vi "BeginService.vi"(1 "In":i32) -> (0 "Out":i32)   [LabVIEW 2011]
doc: "Copyright (c) 2005, Kuan Chen\nAll rights reserved.\n\nRedistribution and use in source and binary forms, with or without modification, are permitted provided that the following conditions are met:\n\n * Redistributions of source code must retain the above copyright notice, this list of conditions and the following disclaimer.\n * Redistributions in binary form must reproduce the above copyright notice, this list of conditions and the following disclaimer in the documentation and/or other materials provided with the distribution.\n * Neither the name of the Kuan Chen nor the names of its contributors may be used to endorse or promote products derived from this software without specific prior written permission.\n\nTHIS SOFTWARE IS PROVIDED BY THE COPYRIGHT HOLDERS AND CONTRIBUTORS \"AS IS\" AND ANY EXPRESS OR IMPLIED WARRANTIES, INCLUDING, BUT NOT LIMITED TO, THE IMPLIED WARRANTIES OF MERCHANTABILITY AND FITNESS FOR A PARTICULAR PURPOSE ARE DISCLAIMED. IN NO EVENT SHALL THE COPYRIGHT OWNER OR CONTRIBUTORS BE LIABLE FOR ANY DIRECT, INDIRECT, INCIDENTAL, SPECIAL, EXEMPLARY, OR CONSEQUENTIAL DAMAGES (INCLUDING, BUT NOT LIMITED TO, PROCUREMENT OF SUBSTITUTE GOODS OR SERVICES; LOSS OF USE, DATA, OR PROFITS; OR BUSINESS INTERRUPTION) HOWEVER CAUSED AND ON ANY THEORY OF LIABILITY, WHETHER IN CONTRACT, STRICT LIABILITY, OR TORT (INCLUDING NEGLIGENCE OR OTHERWISE) ARISING IN ANY WAY OUT OF THE USE OF THIS SOFTWARE, EVEN IF ADVISED OF THE POSSIBILITY OF SUCH DAMAGE.\n\nWrites a \"line n\" line to C:\\temp\\output.txt once per second, where n is the nth second. Stops when StopOutputThread.vi is used."
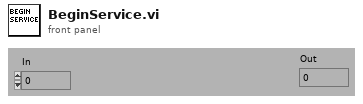
[diagram p1: front panel]
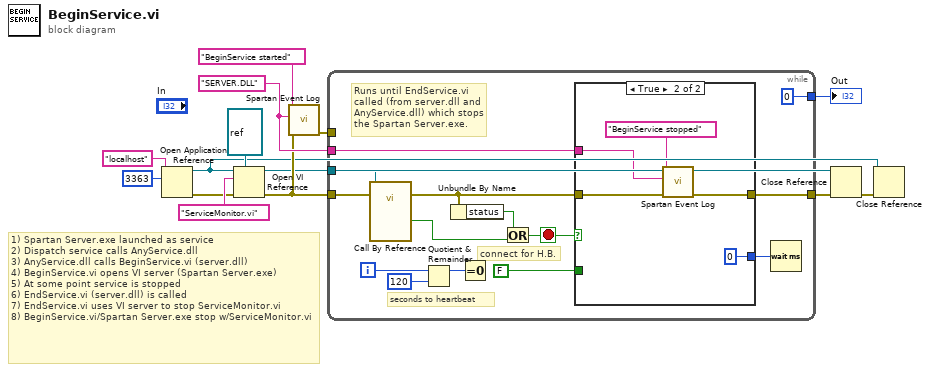
[diagram p0: block diagram]
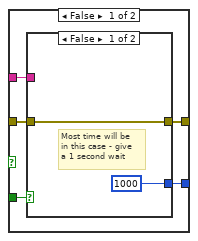
[diagram p2: hidden frame]
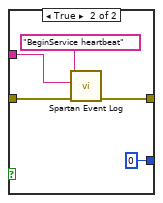
[diagram p3: hidden frame]
diagram:
  w12 = "SERVER.DLL" ("module (\"\")")
  # "1) Spartan Server.exe launched as service\n2) Dispatch service calls AnyService.dll\n3) AnyService.dll calls BeginService.vi (server.dll)\n4) BeginService.vi opens VI server (Spartan Server.exe)\n5) At some point service is stopped\n6) EndService.vi (server.dll) is called\n7) EndService.vi uses VI server to stop ServiceMonitor.vi\n8) BeginService.vi/Spartan Server.exe stop w/ServiceMonitor.vi"
  n1 = Open Application Reference(10:u16 3363 ("port number or service name (3363)"), 11:"localhost" ("machine name (\"\":  open local reference)")) -> (0:w5:errorcluster, 3:w3:refnum<vi>)  [unwired: 2 in]
  n2 = Open VI Reference(type specifier VI Refnum (for type only)=refnum<vi> refnum, application reference (local)=w3, vi path="ServiceMonitor.vi" ("module (\"\")"), error in (no error)=w5) -> (vi reference=w7:refnum<vi>, error out=w10:errorcluster)  [unwired: 2 in]
  n3 = call "Spartan Event Log.vi"("error in (no error)"=w10, "module (\"\")"=w12, "message (\"\")"="BeginService started" ("name (unnamed)")) -> ("error out"=w9:errorcluster)  [unwired: 2 in, 3 out]
  n4 = while {
    tunnel: [0 ("Out")] -> w14
    tunnel: w12 -> [w25]
    tunnel: w10 -> [w21]
    tunnel: w9 -> [_]
    tunnel: w7 -> [w19]
    tunnel: [w17] -> w8
    i -> [w24]
    stop <- w26 stop-if-true
    # "connect for H.B."
    # "seconds to heartbeat"
    # "Runs until EndService.vi\ncalled (from server.dll and\nAnyService.dll) which stops\nthe Spartan Server.exe."
    n5 = call-by-ref "?"(reference=w19, error in=w21) -> (error out=w20:errorcluster, "Stop?"=w18:bool)  [unwired: 1 in, 1 out]
    n6 = Quotient & Remainder(x=w24, y=120) -> (x-y*floor(x/y)=w22:i32)  [unwired: 1 out]
    n7 = Unbundle By Name(w20) -> ("status"=w27:bool)
    n8 = Equal To 0?(x=w22) -> ()  [unwired: 1 out]
    n9 = Or(x=w27, y=w18) -> (x .or. y?=w26:bool)
    n10 = case shown="True" w26 {
      tunnel: w20 -> [w33 w44]
      tunnel: w25 -> [w31 w43]
      tunnel: FALSE -> [w32 _]
      tunnel: [w30 w42] -> w17
      tunnel: [w29 u32 0 ("milliseconds to wait")] -> w15
      frame False {
        n11 = case shown="False" w32 {
          tunnel: w33 -> [w35 w39]
          tunnel: w31 -> [_ w38]
          tunnel: [w35 w37] -> w30
          tunnel: [u32 1000 ("milliseconds to wait") u32 0 ("milliseconds to wait")] -> w29
          frame False {
            # "Most time will be\nin this case - give\na 1 second wait"
          }
          frame True {
            n12 = call "Spartan Event Log.vi"("error in (no error)"=w39, "module (\"\")"=w38, "message (\"\")"="BeginService heartbeat" ("name (unnamed)")) -> ("error out"=w37:errorcluster)  [unwired: 2 in, 3 out]
          }
        }
      }
      frame True {
        n13 = call "Spartan Event Log.vi"("error in (no error)"=w44, "module (\"\")"=w43, "message (\"\")"="BeginService stopped" ("name (unnamed)")) -> ("error out"=w42:errorcluster)  [unwired: 2 in, 3 out]
      }
    }
    n14 = Wait (ms)(milliseconds to wait=w15) -> ()  [unwired: 1 out]
  }
  "Out" <- w14
  n15 = Close Reference(reference=w7, error in (no error)=w8) -> (error out=w4:errorcluster)
  n16 = Close Reference(reference=w3, error in (no error)=w4) -> ()  [unwired: 1 out]
